vi "图片重叠合并.vi"(8 "图片2":picture, 11 "图片1":picture) -> (0 "重叠图片数据":T1 caption="输出簇-合成", 3 "重叠图片":picture)   [LabVIEW 2013]
uses:
  <vilib>/picture/picture.llb/imagedata.ctl
panel:
  out "十六进制颜色":string
  out "Color":u32(colorbox) caption="颜色"
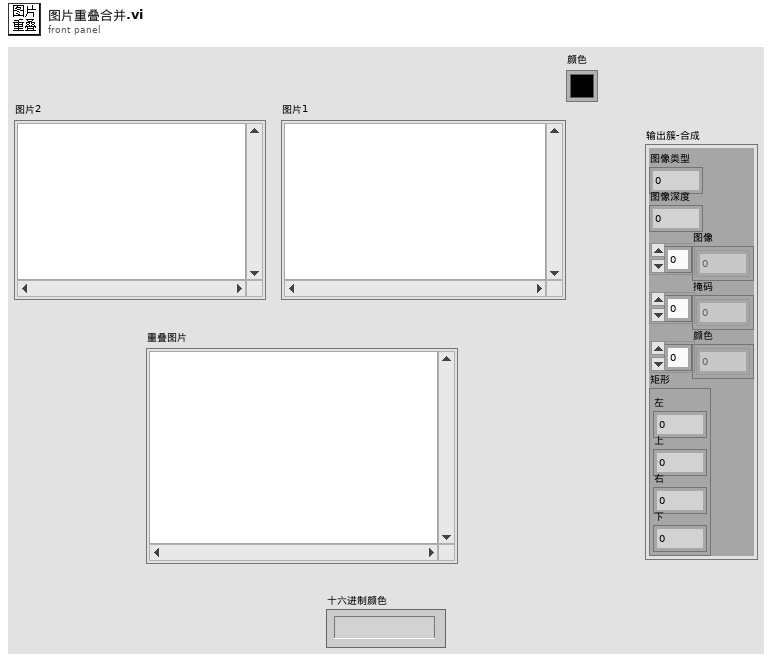
[diagram p1: front panel]
types:
  T1 = typedef "imagedata.ctl" = cluster{"image type":i32, "image depth":i32, "image":u8[], "mask":u8[], "colors":u32[], "Rectangle":cluster{"left":i16, "top":i16, "right":i16, "bottom":i16}}
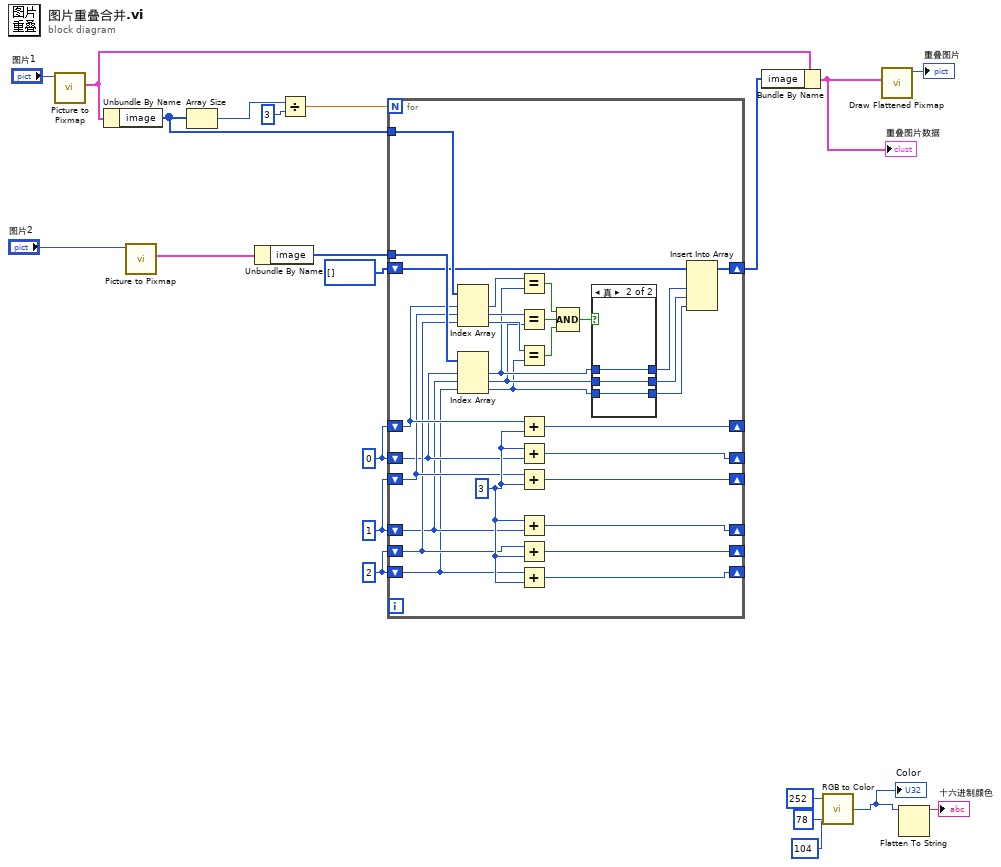
[diagram p0: block diagram]
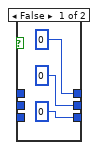
[diagram p2: hidden frame]
diagram:
  w17 = 2
  w18 = 1
  w19 = 0
  n1 = call <vilib>:"Picture to Pixmap.vi"("picture"="图片1") -> ("image data"=w11:T1)  [unwired: 9 in, 1 out]
  n2 = Unbundle By Name(w11) -> ("image"=w16:u8[])
  n3 = call <vilib>:"Picture to Pixmap.vi"("picture"="图片2") -> ("image data"=w21:T1)  [unwired: 9 in, 1 out]
  n4 = Array Size(array=w16) -> (size(s)=w15:i32)
  n5 = Unbundle By Name(w21) -> ("image"=w20:u8[])
  n6 = Divide(x=w15, y=3) -> (x/y=w13:dbl)
  n7 = for {
    N: w13 -> [_]
    tunnel: w16 -> [w51]
    tunnel: w20 -> [w50]
    shift-right: [w49] -> _
    shift-left: w19 -> [w39]
    shift-right: [w46] -> _
    shift-left: w19 -> [w33]
    shift-right: [w45] -> _
    shift-left: w18 -> [w32]
    shift-right: [w44] -> _
    shift-left: w17 -> [w31]
    shift-right: [w47] -> _
    shift-left: w17 -> [w35]
    shift-right: [w48] -> _
    shift-left: w18 -> [w37]
    shift-right: [w29] -> w10
    shift-left: u8[] [] ("image") -> [w30]
    w43 = 3 ("y")
    n8 = Index Array(array=w51, index #1=w39, index #2=w37, index #3=w35) -> (element #1=w38:u8, element #2=w36:u8, element #3=w34:u8)
    n9 = Index Array(array=w50, index #1=w33, index #2=w32, index #3=w31) -> (element #1=w27:u8, element #2=w26:u8, element #3=w22:u8)
    n10 = Equal?(x=w38, y=w27) -> (x = y?=w42:bool)
    n11 = Equal?(x=w36, y=w26) -> (x = y?=w41:bool)
    n12 = Equal?(x=w34, y=w22) -> (x = y?=w40:bool)
    n13 = Add(x=w39, y=w43) -> (x+y=w49:i32)
    n14 = Add(x=w43, y=w33) -> (x+y=w46:i32)
    n15 = Add(x=w37, y=w43) -> (x+y=w48:i32)
    n16 = Add(x=w43, y=w32) -> (x+y=w45:i32)
    n17 = Add(x=w35, y=w43) -> (x+y=w47:i32)
    n18 = Add(x=w31, y=w43) -> (x+y=w44:i32)
    n19 = Compound Arithmetic op=AND(w42, w41, w40) -> (w28:bool)
    n20 = case shown="真" w28 {
      tunnel: w27 -> [_ w57]
      tunnel: w26 -> [_ w56]
      tunnel: w22 -> [_ w55]
      tunnel: [u8 0 w57] -> w25
      tunnel: [u8 0 w56] -> w24
      tunnel: [u8 0 w55] -> w23
      frame False {
      }
      frame True {
      }
    }
    n21 = Insert Into Array(array=w30, new element #1=w25, new element #2=w24, new element #3=w23) -> (w29:u8[])  [unwired: 1 in]
  }
  n22 = Bundle By Name(cluster=w11, "image"=w10) -> (w9:T1)
  "重叠图片数据" <- w9
  n23 = call <vilib>:"RGB to Color.vi"("B"=u8 104, "G"=u8 78, "R"=u8 252) -> ("Color"=w2:u32)
  "Color" <- w2
  n24 = call <vilib>:"Draw Flattened Pixmap.vi"("image data"=w9) -> ("new picture"=→"重叠图片":picture)  [unwired: 8 in]
  n25 = Flatten To String(anything=w2) -> (data string=→"十六进制颜色":string)  [unwired: 3 in, 2 out]
